vi "FP_Get All Controls and Names.vi"(8 "Error":errorcluster, 11 "Generics":refnum<vi>[](array[refnum])) -> (0 "Error Out":errorcluster, 2 "Names Out":string[](array[string]), 3 "Controls[] Out":refnum<vi>[](array[refnum]))   [LabVIEW 2015]
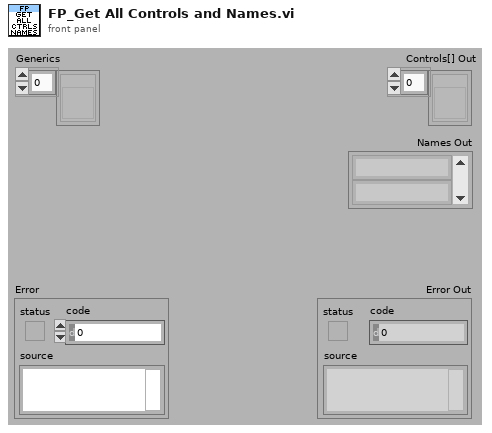
[diagram p1: front panel]
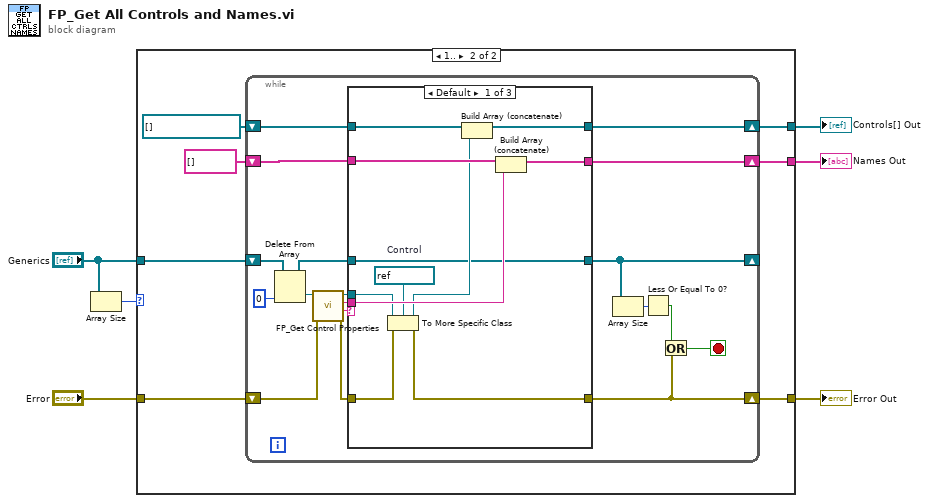
[diagram p0: block diagram]
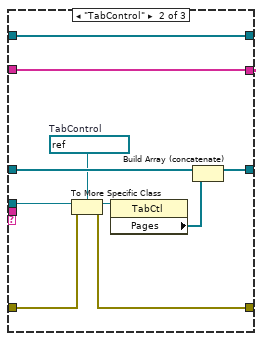
[diagram p3: hidden frame]
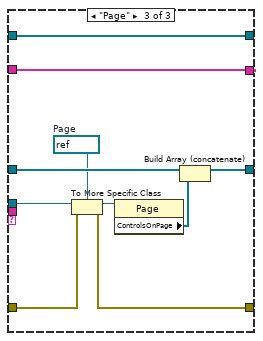
[diagram p4: hidden frame]
diagram:
  n1 = Array Size(array="Generics") -> (size(s)=w3:i32)
  n2 = case shown="1.." w3 {
    tunnel: "Error" -> [w7 w14]
    tunnel: [w7 w13] -> w5
    tunnel: "Generics" -> [_ w12]
    tunnel: [_ w9] -> w2
    tunnel: [_ w8] -> w1
    frame ..0 {
    }
    frame 1.. {
      n3 = while {
        shift-right: [w29] -> _
        shift-left: w12 -> [w32]
        shift-right: [w16] -> w13
        shift-left: w14 -> [w20]
        shift-right: [w24] -> w9
        shift-left: refnum<vi>[] [] -> [w23]
        shift-right: [w22] -> w8
        shift-left: string[] [] -> [w21]
        stop <- w15 stop-if-true
        n4 = Delete From Array(array=w32, index=0) -> (deleted portion=w30:refnum<vi>, array with subset deleted=w28:refnum<vi>[])  [unwired: 1 in]
        n5 = call "FP_Get Control Properties.vi"("Error"=w20, "Ctrl"=w30) -> ("Error Out"=w19:errorcluster, "ClassName Out"=w27:string, "Label.Text Out"=w26:string, "Ctl Refnum Out"=w25:refnum<vi>)  [unwired: 6 in]
        n6 = case shown="Default" w27 {
          tunnel: w28 -> [w35 w53 w63]
          tunnel: [w35 w50 w60] -> w29
          tunnel: w26 -> [w41 _ _]
          tunnel: w25 -> [w38 w49 w59]
          tunnel: [w43 w51 w61] -> w24
          tunnel: w23 -> [w42 w51 w61]
          tunnel: [w40 w52 w62] -> w22
          tunnel: w21 -> [w39 w52 w62]
          tunnel: w19 -> [w34 w48 w58]
          tunnel: [w33 w47 w57] -> w16
          frame Default {
            w36 = refnum<vi> refnum  # Control
            n7 = To More Specific Class(target class=w36, reference=w38, error in=w34) -> (specific class reference=w37:refnum<vi>, error out=w33:errorcluster)
            n8 = Build Array (concatenate)(w42, w37) -> (w43:refnum<vi>[])
            n9 = Build Array (concatenate)(w39, w41) -> (w40:string[])
          }
          frame "TabControl" {
            w45 = refnum<vi> refnum  # TabControl
            n10 = To More Specific Class(target class=w45, reference=w49, error in=w48) -> (specific class reference=w46:refnum<vi>, error out=w47:errorcluster)
            n11 = property class="TabCtl"(reference=w46) -> ("Pages"=w44:refnum<vi>[])  [unwired: 1 in, 2 out]
            n12 = Build Array (concatenate)(w53, w44) -> (w50:refnum<vi>[])
          }
          frame "Page" {
            w55 = refnum<vi> refnum  # Page
            n13 = To More Specific Class(target class=w55, reference=w59, error in=w58) -> (specific class reference=w56:refnum<vi>, error out=w57:errorcluster)
            n14 = property class="Page"(reference=w56) -> ("ControlsOnPage"=w54:refnum<vi>[])  [unwired: 1 in, 2 out]
            n15 = Build Array (concatenate)(w63, w54) -> (w60:refnum<vi>[])
          }
        }
        n16 = Array Size(array=w29) -> (size(s)=w31:i32)
        n17 = Less Or Equal To 0?(x=w31) -> (x <= 0?=w17:bool)
        n18 = Or(x=w17, y=w16) -> (x .or. y?=w15:bool)
      }
    }
  }
  "Controls[] Out" <- w2
  "Error Out" <- w5
  "Names Out" <- w1
